vi "Display.vi"(8 "error in (no error)":errorcluster, 11 "Solartron in":refnum<class "Solartron.lvclass">) -> (0 "error out":errorcluster, 3 "Solartron out":refnum<class "Solartron.lvclass">)   [LabVIEW 2014, in "Solartron.lvlib" / "Solartron.lvclass"]
uses:
  Solartron.lvclass
panel:
  out "Transductor 4":dbl(slide) scale=0.0..1.0
  out "Transductor 3":dbl(slide) scale=0.0..1.0
  out "Transductor 2":dbl(slide) scale=0.0..1.0
  out "Transductor 1":dbl(slide) scale=0.0..1.0
  in  "STOP":bool
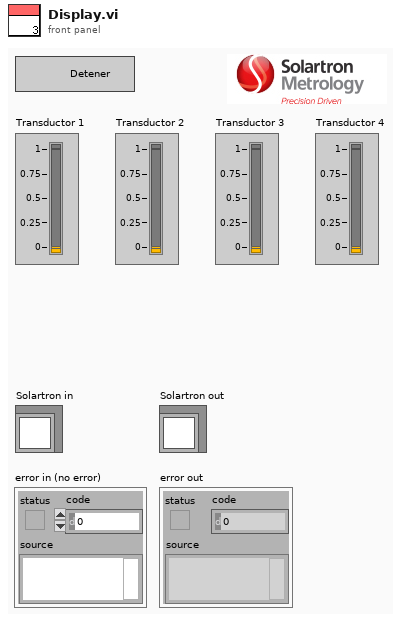
[diagram p1: front panel]
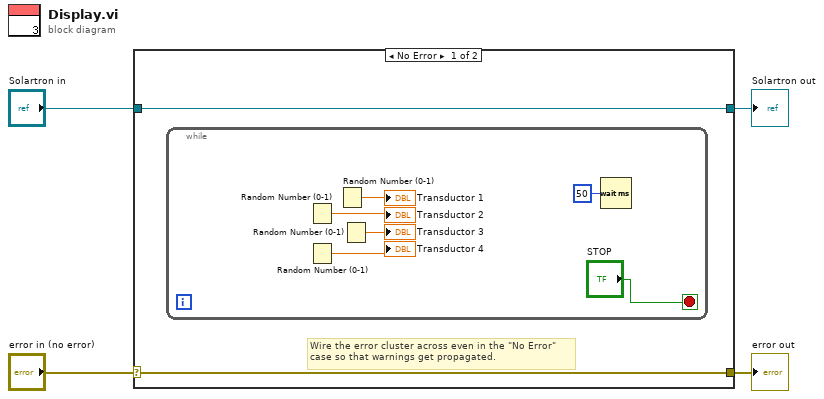
[diagram p0: block diagram]
diagram:
  n1 = case shown="No Error" "error in (no error)" {
    selector: "error in (no error)" -> [w5 w14]
    tunnel: [w5 w14] -> w3
    tunnel: [w6 w13] -> w1
    tunnel: "Solartron in" -> [w6 w13]
    frame No Error {
      # "Wire the error cluster across even in the \"No Error\"\ncase so that warnings get propagated."
      n2 = while {
        stop <- "STOP" stop-if-true
        n3 = Random Number (0-1)() -> (number: 0 to 1=→"Transductor 2":dbl)
        n4 = Random Number (0-1)() -> (number: 0 to 1=→"Transductor 4":dbl)
        n5 = Random Number (0-1)() -> (number: 0 to 1=→"Transductor 1":dbl)
        n6 = Random Number (0-1)() -> (number: 0 to 1=→"Transductor 3":dbl)
        n7 = Wait (ms)(milliseconds to wait=u32 50) -> ()  [unwired: 1 out]
      }
    }
    frame Error {
    }
  }
  "error out" <- w3
  "Solartron out" <- w1
